vi "Create Default Channel.vi"(7 "URL":T3, 8 "channel classification":T1, 9 "data type":T2, 10 "variable name":string, 11 "hostname":string="localhost") -> (3 "channel":refnum<class "TBM channel.lvclass">)   [LabVIEW 2013, in "Scan Engine configuration.lvclass"]
uses:
  Scan Engine configuration.lvclass
  Protocol.ctl
  <vilib>/NI/Tag Bus Module Framework/channel/TBM channel.lvclass
  <vilib>/NI/Tag Bus/tag/Data Type.ctl
  <vilib>/NI/Tag Bus Module Framework/channel/channel classification.ctl
  <vilib>/NI/Tag Bus/tag/tag descriptor.lvclass
  editor node/Scan Engine editor node.lvclass
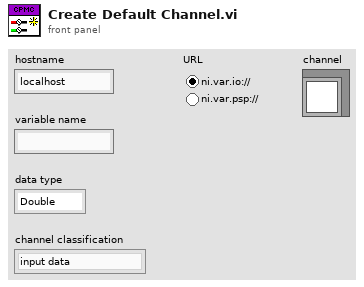
[diagram p1: front panel]
types:
  T1 = typedef "TBM channel.lvclass/channel classification.ctl" = enum16{"input data", "output data", "processing parameter", "processing result"}
  T2 = typedef "tag bus.lvlib/tag descriptor.lvclass/Data Type.ctl" = enum16{"Double", "Single", "I64", "I32", "I16", "I8", "U64", "U32", "U16", "U8", "Boolean", "String", "Array of Double", "Array of Single", "Array of I64", "Array of I32", "Array of I16", "Array of I8", "Array of U64", "Array of U32", "Array of U16", "Array of U8", "Array of Boolean", "Array of String"}
  T3 = typedef "Scan Engine editor node.lvclass/Protocol.ctl" = enum32{"ni.var.io://", "ni.var.psp://"}
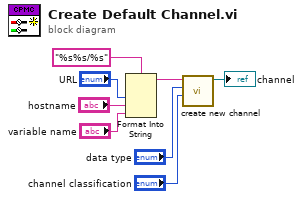
[diagram p0: block diagram]
diagram:
  n1 = Format Into String(format string="%s%s/%s", "URL", "hostname", "variable name") -> (resulting string=w3:string)  [unwired: 2 in, 1 out]
  n2 = call <vilib>:"create new channel.vi"("channel classification"="channel classification", "data type"="data type", "channel name"=w3) -> ("channel"=→"channel":refnum<class "TBM channel.lvclass">)  [unwired: 8 in]
